vi "userROI.vi"(6 "Numeric":i32, 9 "Command":string, 10 "Channel":string, 11 "CamSettings in":T1) -> (2 "before substring":string, 3 "CamSettings out":T1)   [LabVIEW 2020]
uses:
  CamSettings_Typdef.ctl
  CamSettingSUB_TypDEf.ctl
  CamAndObj_TypDEf.ctl
  OnOffTypeDef.ctl
  userROI.ctl
  source/Device Drivers/shared/numericVariable_TypeDef.ctl
  CamRoiTypDef.ctl
  source/Device Drivers/BaseDriver/BaseDriver.lvclass
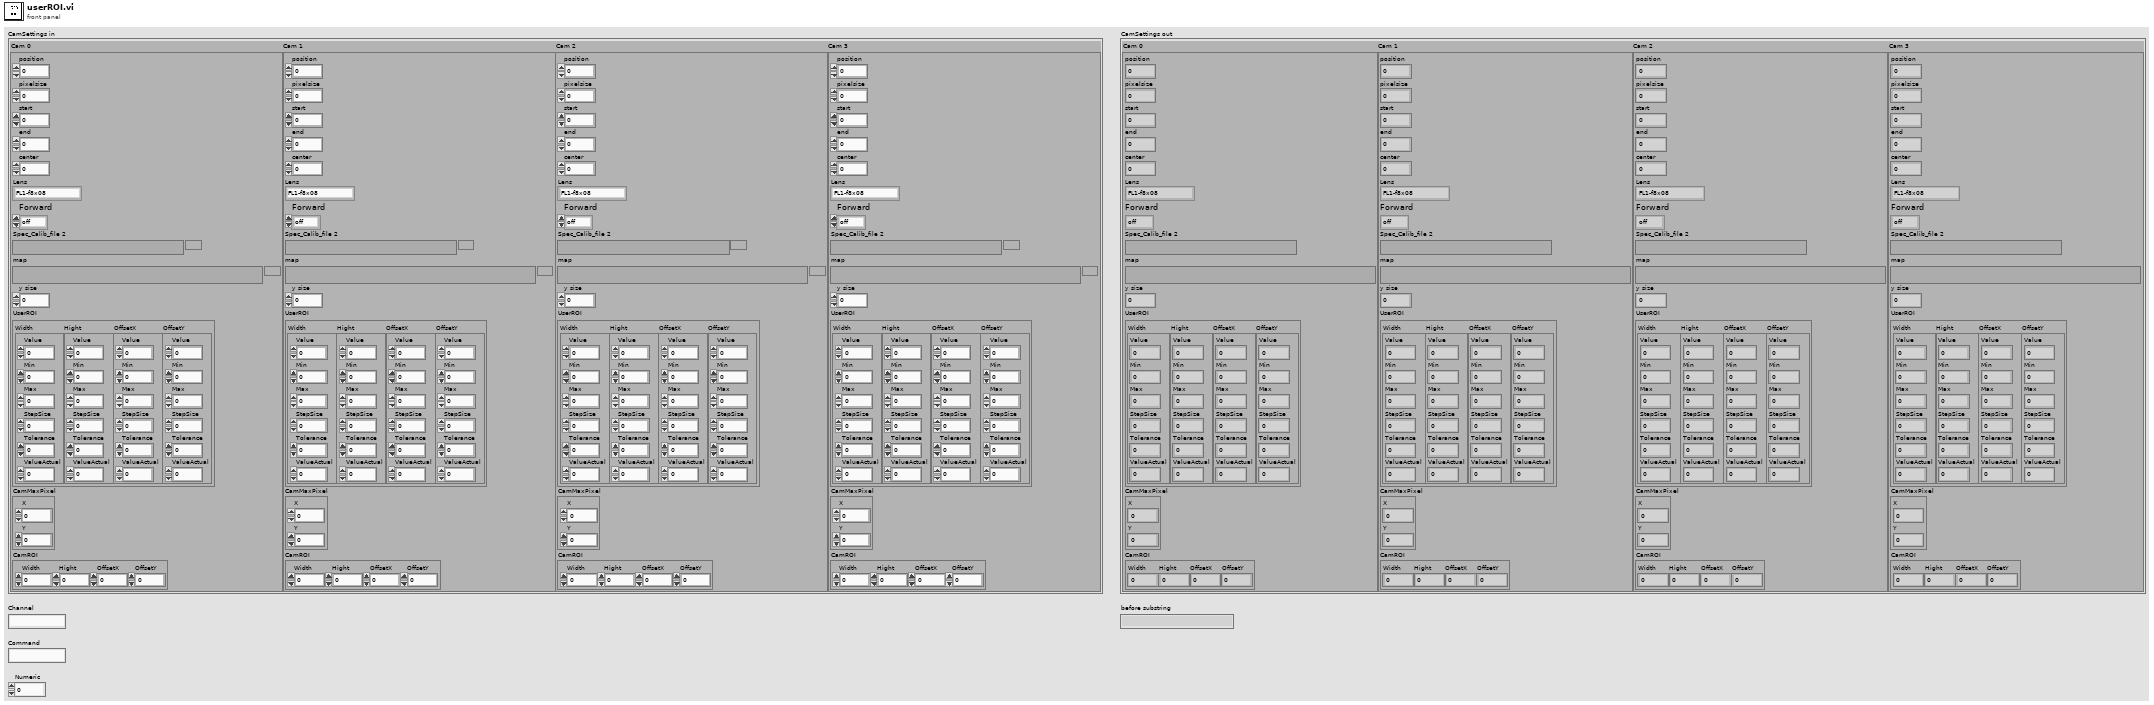
[diagram p1: front panel]
types:
  T1 = typedef "CamSettings_Typdef.ctl" = cluster{"Cam 0":T2, "Cam 1":T2, "Cam 2":T2, "Cam 3":T2}
  T2 = typedef "CamSettingSUB_TypDEf.ctl" = cluster{"position":dbl, "pixelsize":dbl, "start":dbl, "end":dbl, "center":dbl, "Lens":T3, "Forward":T4, "Spec_Calib_file 2":path, "map":path, "y size":i32, "UserROI":T5, "CamMaxPixel":cluster{"X":i32, "Y":i32}, "CamROI":T7}
  T3 = typedef "CamAndObj_TypDEf.ctl" = enum16{"FL1-f8x08", "FL1-f8x06", "FL1-f8", "ch300-f50", "FL2G-f8", "FL3M14-f8", "FL3M14-f8x08", "FL3M14-f8x08(2x2)"}
  T4 = typedef "OnOffTypeDef.ctl" = enum16{"off", "on"}
  T5 = typedef "userROI.ctl" = cluster{"Width":T6, "Hight":T6, "OffsetX":T6, "OffsetY":T6}
  T6 = typedef "BaseDriver.lvclass/numericVariable_TypeDef.ctl" = cluster{"Value":dbl, "Min":dbl, "Max":dbl, "StepSize":dbl, "Tolerance":dbl, "ValueActual":dbl}
  T7 = typedef "CamRoiTypDef.ctl" = cluster{"Width":dbl, "Hight":dbl, "OffsetX":dbl, "OffsetY":dbl}
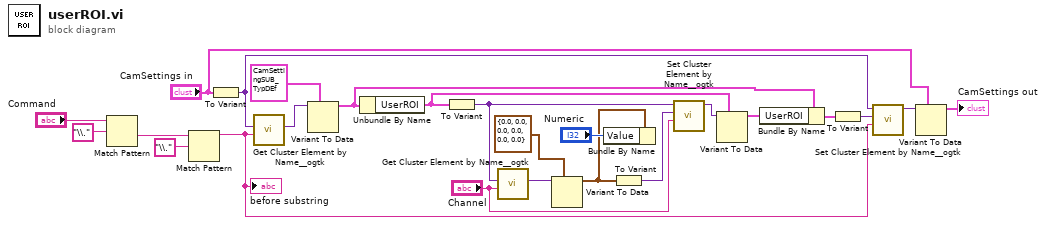
[diagram p0: block diagram]
diagram:
  n1 = Match Pattern(string="Command", regular expression="\\.") -> (after substring=w7:string)  [unwired: 1 in, 3 out]
  n2 = Match Pattern(string=w7, regular expression="\\.") -> (before substring=w13:string)  [unwired: 1 in, 3 out]
  "before substring" <- w13
  n3 = To Variant(anything="CamSettings in") -> (Variant=w12:variant)
  n4 = call "Get Cluster Element by Name__ogtk.vi"("Element Name"=w13, "Cluster"=w12) -> ("VElement"=w8:variant)  [unwired: 7 in, 2 out]
  n5 = Variant To Data(type=T2 {"position"=0.0, "pixelsize"=0.0, "start"=0.0, "end"=0.0, "center"=0.0, "Lens"=enum."FL1-f8x08", "Forward"=enum."off", "Spec_Calib_file 2"=path "Y:/100TWdata/ESMCalib/datFwd.txt", "map"=path "Y:/100TWdata/ESMCalib/mapFwd.txt", "y size"=0, "UserROI"={"Width"={"Value"=0.0, "Min"=0.0, "Max"=0.0, "StepSize"=0.0, "Tolerance"=0.0, "ValueActual"=0.0}, "Hight"={"Value"=0.0, "Min"=0.0, "Max"=0.0, "StepSize"=0.0, "Tolerance"=0.0, "ValueActual"=0.0}, "OffsetX"={"Value"=0.0, "Min"=0.0, "Max"=0.0, "StepSize"=0.0, "Tolerance"=0.0, "ValueActual"=0.0}, "OffsetY"={"Value"=0.0, "Min"=0.0, "Max"=0.0, "StepSize"=0.0, "Tolerance"=0.0, "ValueActual"=0.0}}, "CamMaxPixel"={"X"=0, "Y"=0}, "CamROI"={"Width"=0.0, "Hight"=0.0, "OffsetX"=0.0, "OffsetY"=0.0}} ("Cam 0"), Variant=w8) -> (data=w23:T2)  [unwired: 1 in, 1 out]
  n6 = Unbundle By Name(w23) -> ("UserROI"=w10:T5)
  n7 = To Variant(anything=w10) -> (Variant=w17:variant)
  n8 = call "Get Cluster Element by Name__ogtk.vi"("Element Name"="Channel", "Cluster"=w17) -> ("VElement"=w19:variant)  [unwired: 7 in, 2 out]
  n9 = Variant To Data(type=T6 {"Value"=0.0, "Min"=0.0, "Max"=0.0, "StepSize"=0.0, "Tolerance"=0.0, "ValueActual"=0.0} ("Width"), Variant=w19) -> (data=w4:T6)  [unwired: 1 in, 1 out]
  n10 = Bundle By Name(cluster=w4, "Value"="Numeric") -> ()  [unwired: 1 out]
  n11 = To Variant(anything=w4) -> (Variant=w3:variant)
  n12 = call "Set Cluster Element by Name__ogtk.vi"("Element Name (\"\": New Element Data Name)"="Channel", "New Element Value"=w3, "Cluster"=w17) -> ("VCluster out"=w9:variant)  [unwired: 6 in, 2 out]
  n13 = Variant To Data(type=w10, Variant=w9) -> (data=w11:T5)  [unwired: 1 in, 1 out]
  n14 = Bundle By Name(cluster=w23, "UserROI"=w11) -> (w2:T2)
  n15 = To Variant(anything=w2) -> (Variant=w1:variant)
  n16 = call "Set Cluster Element by Name__ogtk.vi"("Element Name (\"\": New Element Data Name)"=w13, "New Element Value"=w1, "Cluster"=w12) -> ("VCluster out"=w14:variant)  [unwired: 6 in, 2 out]
  n17 = Variant To Data(type="CamSettings in", Variant=w14) -> (data=→"CamSettings out":T1)  [unwired: 1 in, 1 out]
